vi "4 Ch Digital Output.vi"(2 "Packet":u64, 4 "4 Ch Digital Out":T1={"DO0"="NI 9474/DO0", "DO1"="NI 9474/DO1", "DO2"="NI 9474/DO2", "DO3"="NI 9474/DO3"}) -> ()   [LabVIEW 2010]
uses:
  <vilib>/eio/EIONode/EIONode.xnode
  <vilib>/rvi/eio/nirviEIOImplementation/nirviEIOImplementation.xnode
  <vilib>/rvi/eio/common/nirviEmuClasses.ctl
  <vilib>/rvi/eio/common/nirviEmuTemplateMethod_noerrors.vi
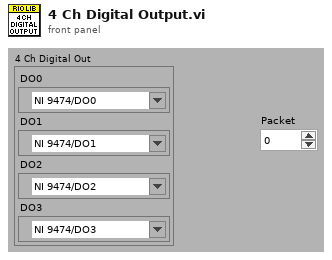
[diagram p1: front panel]
types:
  T1 = cluster{"DO0":refnum<k21>, "DO1":refnum<k21>, "DO2":refnum<k21>, "DO3":refnum<k21>}
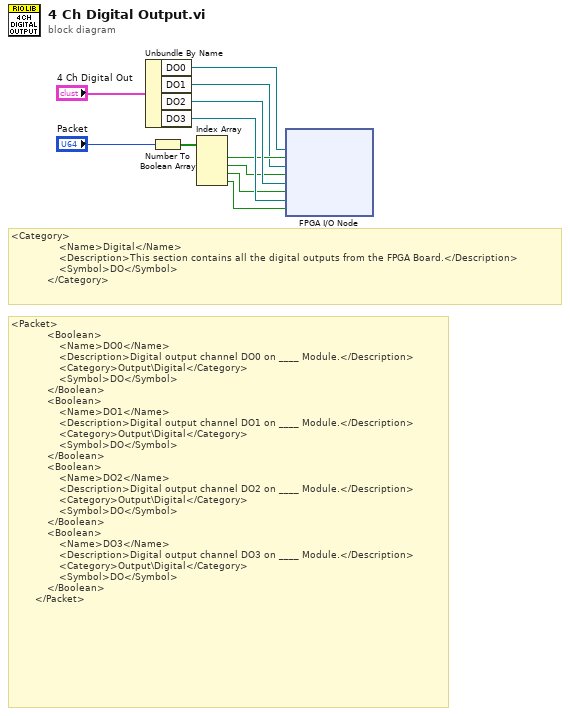
[diagram p0: block diagram]
diagram:
  # "<Category>\n                <Name>Digital</Name>\n                <Description>This section contains all the digital outputs from the FPGA Board.</Description>\n                <Symbol>DO</Symbol>\n            </Category>"
  # "<Packet>\n            <Boolean>\n                <Name>DO0</Name>\n                <Description>Digital output channel DO0 on ____ Module.</Description>\n                <Category>Output\\Digital</Category>\n                <Symbol>DO</Symbol>\n            </Boolean>\n            <Boolean>\n                <Name>DO1</Name>\n                <Description>Digital output channel DO1 on ____ Module.</Description>\n                <Category>Output\\Digital</Category>\n                <Symbol>DO</Symbol>\n            </Boolean>\n            <Boolean>\n                <Name>DO2</Name>\n                <Description>Digital output channel DO2 on ____ Module.</Description>\n                <Category>Output\\Digital</Category>\n                <Symbol>DO</Symbol>\n            </Boolean>\n            <Boolean>\n                <Name>DO3</Name>\n                <Description>Digital output channel DO3 on ____ Module.</Description>\n                <Category>Output\\Digital</Category>\n                <Symbol>DO</Symbol>\n            </Boolean>\n        </Packet>"
  n1 = Unbundle By Name("4 Ch Digital Out") -> ("DO0"=w2:refnum<k21>, "DO1"=w1:refnum<k21>, "DO2"=w11:refnum<k21>, "DO3"=w10:refnum<k21>)
  n2 = Number To Boolean Array(number="Packet") -> (Boolean array=w4:bool[])
  n3 = Index Array(array=w4) -> (element #1=w5:bool, element #2=w8:bool, element #3=w7:bool, element #4=w6:bool)  [unwired: 4 in]
  n4 = xnode "FPGA I/O Node"("I/O Item"=w5, "I/O Item"=w8, "I/O Item"=w7, "I/O Item"=w6, "FPGA I/O In"=w2, "FPGA I/O In"=w1, "FPGA I/O In"=w11, "FPGA I/O In"=w10) -> ()  [unwired: 4 out]
